vi "GT Set Pid.vi"(7 "pPid":T1, 8 "error in (no error)":errorcluster caption="错误输入（无错误）", 9 "index":i16, 10 "control":i16, 11 "cardNum":i16) -> (0 "error out":errorcluster caption="错误输出", 3 "function return":i16, 5 "pPid out":T1)   [LabVIEW 2020, in "gts.lvlib"]
doc: "GT_API GT_SetPid(short cardNum,short control,short index,TPid *pPid);"
uses:
  gts.lvlib
  dll/32bit/multi_card/gts.dll
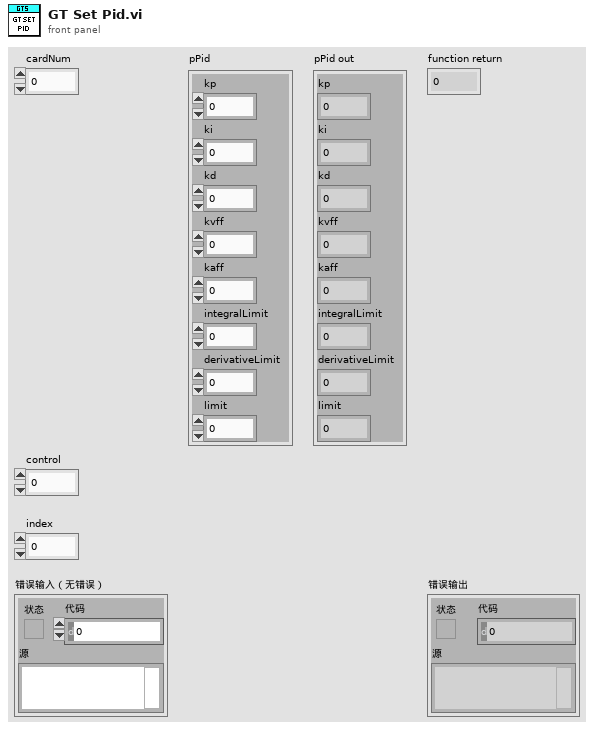
[diagram p1: front panel]
types:
  T1 = cluster{"kp":dbl, "ki":dbl, "kd":dbl, "kvff":dbl, "kaff":dbl, "integralLimit":i32, "derivativeLimit":i32, "limit":i16}
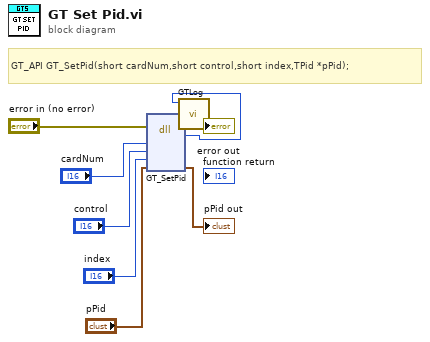
[diagram p0: block diagram]
diagram:
  # "GT_API GT_SetPid(short cardNum,short control,short index,TPid *pPid);"
  n1 = dll-call lib="C:/1228/dll/32bit/multi_card/gts.dll" fn="GT_SetPid"(error in="error in (no error)", "cardNum"="cardNum", "control"="control", "index"="index", "pPid"="pPid") -> (error out=w3:errorcluster, w1:i16, "pPid"=→"pPid out":T1)  [unwired: 5 in, 1 out]
  n2 = call "GTLog.vi"("error in (no error)"=w3, "Numeric"=w1) -> ("error out"=→"error out":errorcluster)  [unwired: 9 in]
